vi "Add DAQ Hardware_Add DAQ.vi"(8 "error in (no error)":errorcluster, 9 "Settings":T1={"Name"="", "Description"="", "InputConfiguration"=10078, "TurnOffHWTimedSinglePointAI"=FALSE, "TurnOffHWTimedSinglePointAO"=FALSE, "DAQConversionRateOption"=0, "PortWidth"=0, "Analog Inputs"=[], "Analog Outputs"=[], "DIO Port Settings"=[], "Counter Settings"={"Frequency Measurements"=[], "Period Measurements"=[], "Count Measurements"=[], "Position Measurements"=[]}} {"Counter Settings"."Position Measurements"."ZIndexMode" items=["AHighBHigh"=10040, "AHighBLow"=10041, "ALowBHigh"=10042, "ALowBLow"=10043]; "Counter Settings"."Position Measurements"."Decoding" items=["Decoding1X"=10090, "Decoding2X"=10091, "Decoding4X"=10092, "DecodingPulseCounting"=10313]; "Counter Settings"."Count Measurements"."CountDirection" items=["Down"=10124, "Up"=10128, "ExternallyControlled"=10326]; "Counter Settings"."Count Measurements"."Edge" items=["Falling"=10171, "Rising"=10280]; "Counter Settings"."Period Measurements"."Edge" items=["Falling"=10171, "Rising"=10280]; "Counter Settings"."Frequency Measurements"."Edge" items=["Falling"=10171, "Rising"=10280]; "Analog Outputs"."ChannelType" items=["Voltage", "Current"]; "Analog Inputs"."ChannelType" items=["Voltage", "Current"]; "DAQConversionRateOption" items=["Default", "Maximum"]; "InputConfiguration" items=["NRSE"=10078, "RSE"=10083, "Differential"=10106, "Pseudodifferential"=12529, "Default"=-1]}, 11 "DAQ Ref":refnum<k24>) -> (0 "error out":errorcluster, 3 "DAQ Ref Out":refnum<k24>)   [LabVIEW 2019, in "Simple SysDef API.lvlib"]
uses:
  <userlib>/SimpleSysDef/Simple SysDef API.lvlib
  <userlib>/SimpleSysDef/_SubVIs/Add DAQ Hardware_Settings.ctl
  <userlib>/SimpleSysDef/_SubVIs/Add DAQ Hardware_Analog Settings.ctl
  <userlib>/SimpleSysDef/_SubVIs/Add DAQ Hardware_Digital Port Settings.ctl
  <userlib>/SimpleSysDef/_SubVIs/Add DAQ Hardware_Digital Settings.ctl
  <userlib>/SimpleSysDef/_SubVIs/Add Frequency Measurement Channels_Settings.ctl
  <userlib>/SimpleSysDef/_SubVIs/Add Count Measurement Channels_Settings.ctl
  NationalInstruments.VeriStand.SystemDefinitionAPI
  <userlib>/SimpleSysDef/_SubVIs/Add Position Measurement Channels_Settings.ctl
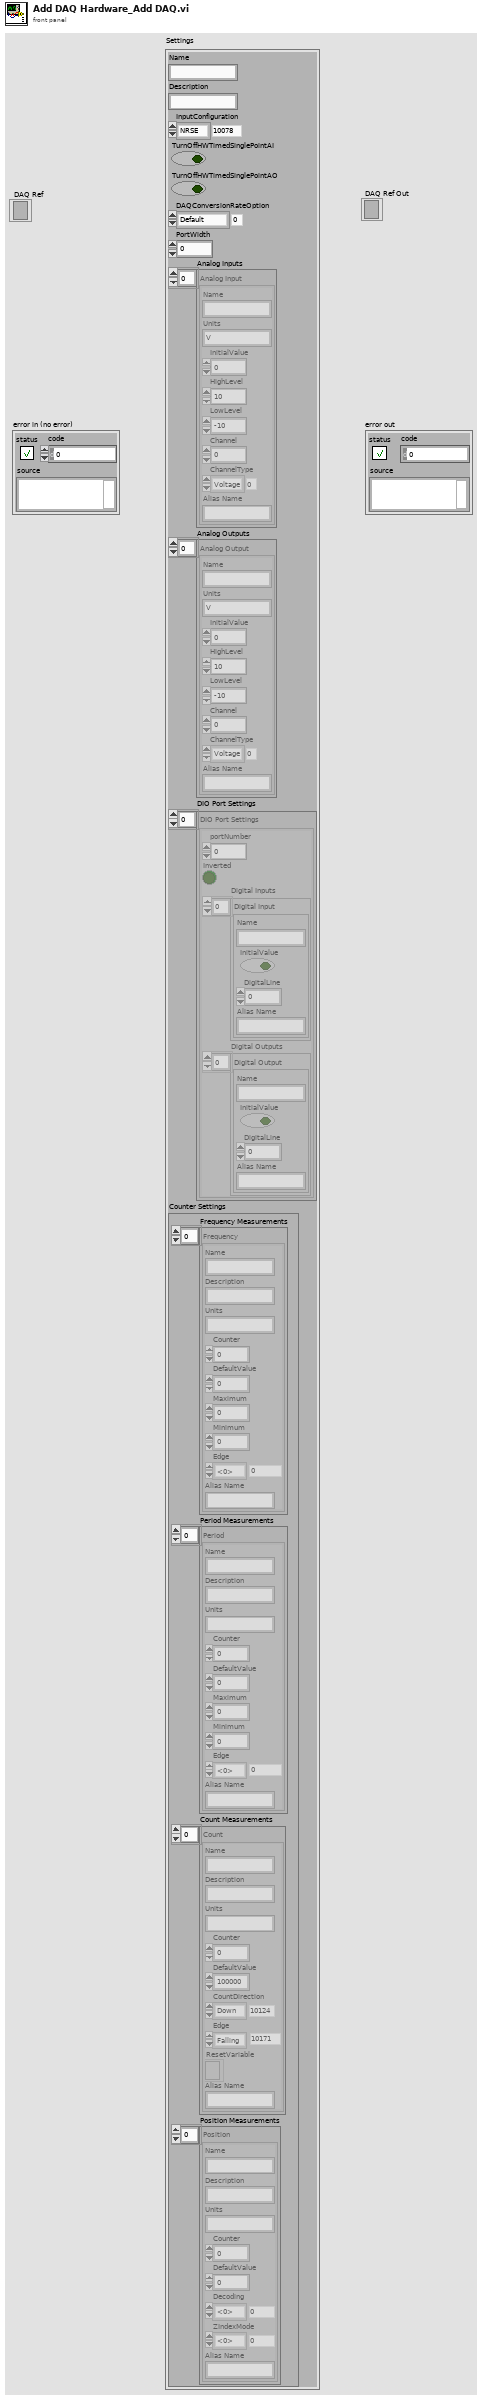
[diagram p1: front panel]
types:
  T1 = typedef "Simple SysDef API.lvlib/Add DAQ Hardware_Settings.ctl" = cluster{"Name":string, "Description":string, "InputConfiguration":i32, "TurnOffHWTimedSinglePointAI":bool, "TurnOffHWTimedSinglePointAO":bool, "DAQConversionRateOption":i32, "PortWidth":u16, "Analog Inputs":T2[], "Analog Outputs":T2[], "DIO Port Settings":T3[], "Counter Settings":cluster{"Frequency Measurements":T5[], "Period Measurements":T5[], "Count Measurements":T6[], "Position Measurements":T7[]}}
  T2 = typedef "Simple SysDef API.lvlib/Add DAQ Hardware_Analog Settings.ctl" = cluster{"Name":string, "Units":string, "InitialValue":dbl, "HighLevel":dbl, "LowLevel":dbl, "Channel":u32, "ChannelType":i32, "Alias Name":string}
  T3 = typedef "Simple SysDef API.lvlib/Add DAQ Hardware_Digital Port Settings.ctl" = cluster{"portNumber":u32, "Inverted":bool, "Digital Inputs":T4[], "Digital Outputs":T4[]}
  T4 = typedef "Simple SysDef API.lvlib/Add DAQ Hardware_Digital Settings.ctl" = cluster{"Name":string, "InitialValue":bool, "DigitalLine":u32, "Alias Name":string}
  T5 = typedef "Simple SysDef API.lvlib/Add Frequency Measurement Channels_Settings.ctl" = cluster{"Name":string, "Description":string, "Units":string, "Counter":u32, "DefaultValue":dbl, "Maximum":dbl, "Minimum":dbl, "Edge":i32, "Alias Name":string}
  T6 = typedef "Simple SysDef API.lvlib/Add Count Measurement Channels_Settings.ctl" = cluster{"Name":string, "Description":string, "Units":string, "Counter":u32, "DefaultValue":dbl, "CountDirection":i32, "Edge":i32, "ResetVariable":refnum<k24>, "Alias Name":string}
  T7 = typedef "Simple SysDef API.lvlib/Add Position Measurement Channels_Settings.ctl" = cluster{"Name":string, "Description":string, "Units":string, "Counter":u32, "DefaultValue":dbl, "Decoding":i32, "ZIndexMode":i32, "Alias Name":string}
  T8 = cluster{"Frequency Measurements":T5[], "Period Measurements":T5[], "Count Measurements":T6[], "Position Measurements":T7[]}
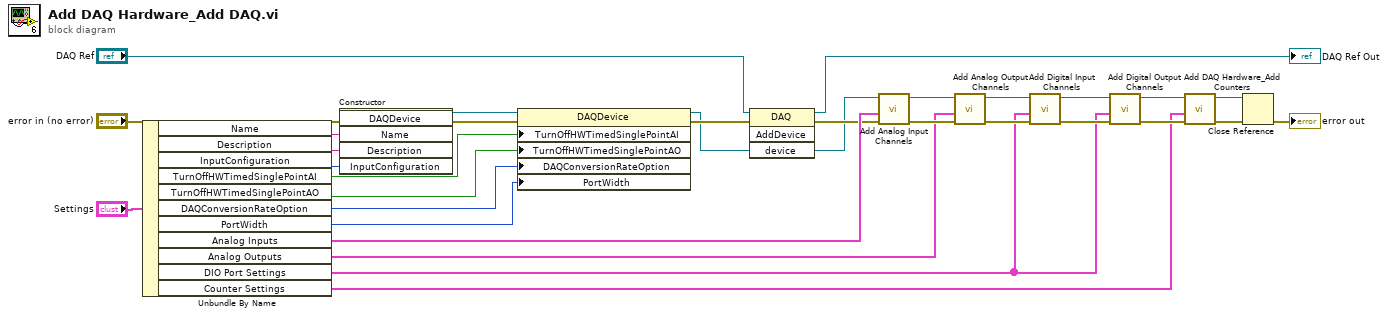
[diagram p0: block diagram]
diagram:
  n1 = Unbundle By Name("Settings") -> ("Name"=w20:string, "Description"=w19:string, "InputConfiguration"=w18:i32, "TurnOffHWTimedSinglePointAI"=w17:bool, "TurnOffHWTimedSinglePointAO"=w16:bool, "DAQConversionRateOption"=w15:i32, "PortWidth"=w14:u16, "Analog Inputs"=w13:T2[], "Analog Outputs"=w12:T2[], "DIO Port Settings"=w11:T3[], "Counter Settings"=w10:T8)
  n2 = constructor class="DAQDevice"(error in="error in (no error)", "Name"=w20, "Description"=w19, "InputConfiguration"=w18) -> (reference out=w31:refnum<k24>, error out=w30:errorcluster)  [unwired: 2 in, 4 out]
  n3 = property class="DAQDevice"(reference=w31, error in=w30, "TurnOffHWTimedSinglePointAI"=w17, "TurnOffHWTimedSinglePointAO"=w16, "DAQConversionRateOption"=w15, "PortWidth"=w14) -> (reference out=w1:refnum<k24>, error out=w5:errorcluster)
  n4 = invoke class="DAQ" method="AddDevice"(reference="DAQ Ref", error in=w5, "device"=w1) -> (reference out=→"DAQ Ref Out":refnum<k24>, error out=w4:errorcluster)  [unwired: 1 in, 2 out]
  n5 = call <userlib>:"Add Analog Input Channels.vi"("error in (no error)"=w4, "Analog Inputs"=w13, "DAQ Ref"=w1) -> ("error out"=w29:errorcluster, "DAQ Ref"=w28:refnum<k24>)  [unwired: 7 in]
  n6 = call <userlib>:"Add Analog Output Channels.vi"("error in (no error)"=w29, "Analog Outputs"=w12, "DAQ Ref"=w28) -> ("error out"=w27:errorcluster, "DAQ Ref"=w25:refnum<k24>)  [unwired: 7 in]
  n7 = call <userlib>:"Add Digital Input Channels.vi"("error in (no error)"=w27, "DIO Port Settings"=w11, "DAQ Ref"=w25) -> ("error out"=w26:errorcluster, "DAQ Ref"=w24:refnum<k24>)  [unwired: 7 in]
  n8 = call <userlib>:"Add Digital Output Channels.vi"("error in (no error)"=w26, "DIO Port Settings"=w11, "DAQ Ref"=w24) -> ("error out"=w23:errorcluster, "DAQ Ref"=w22:refnum<k24>)  [unwired: 7 in]
  n9 = call <userlib>:"Add DAQ Hardware_Add Counters.vi"("error in (no error)"=w23, "Counter Settings"=w10, "DAQ Ref"=w22) -> ("error out"=w6:errorcluster, "DAQ Ref Out"=w9:refnum<k24>)  [unwired: 7 in]
  n10 = Close Reference(reference=w9, error in (no error)=w6) -> (error out=→"error out":errorcluster)
